vi "AddNodePortToGlobal.vi"(3 "ROS in":T1) -> ()   [LabVIEW 2012]
uses:
  <userlib>/ROSforLV/ROS/Code/SubVIs/_ROSControl.ctl
  <userlib>/ROSforLV/ROS/Code/SubVIs/_ROSDirection.ctl
  <userlib>/ROSforLV/ROS/Code/_ROSDefinition.vi
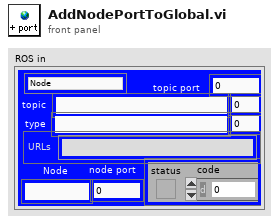
[diagram p1: front panel]
types:
  T1 = typedef "_ROSControl.ctl" = cluster{"topic port":u16, "Node":string, "topic":string, "type":string, "node port":u16, "error ":errorcluster, "Direction":T2, "APIs":string[], "Update (ms)":u16, "write queue":u16}
  T2 = typedef "_ROSDirection.ctl" = enum16{"Node", "Publisher", "Subscriber", "Service Client"}
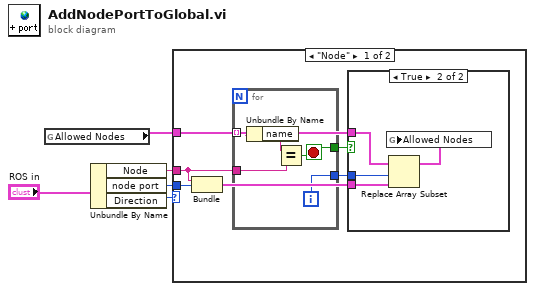
[diagram p0: block diagram]
diagram:
  n1 = global read "_ROSDefinition.vi" "Allowed Nodes"() -> (w3:cluster{"name":string, "Port":u16}[])
  n2 = Unbundle By Name("ROS in") -> ("Node"=w2:string, "node port"=w1:u16, "Direction"=w5:T2)
  n3 = case shown="\"Node\"" w5 {
    tunnel: w3 -> [w8 _]
    tunnel: w2 -> [w9 _]
    tunnel: w1 -> [w10 _]
    frame "Node" {
      n4 = Bundle("Node"=w9, "node port"=w10) -> (w7:cluster{"Node":string, "node port":u16})  [unwired: 1 in]
      n5 = for {
        tunnel: w8 -> [w20] mode=indexing
        tunnel: w9 -> [w18]
        tunnel: [w17] -> w11
        tunnel: [w16] -> w6
        i -> [w16]
        stop <- w17 stop-if-true
        n6 = Unbundle By Name(w20) -> ("name"=w19:string)
        n7 = Equal?(x=w19, y=w18) -> (x = y?=w17:bool)
      }
      n8 = case shown="True" w11 {
        tunnel: w8 -> [_ w15]
        tunnel: w7 -> [_ w14]
        tunnel: w6 -> [_ w13]
        frame False {
        }
        frame True {
          n9 = Replace Array Subset(array=w15, new element=w14, index=w13) -> (w12:cluster{"name":string, "Port":u16}[])
          n10 = global write "_ROSDefinition.vi" "Allowed Nodes"(w12) -> ()
        }
      }
    }
    frame Default {
    }
  }
